vi "Build DAQmx Settings.vi"(7 "Host Resources":T10, 11 "Hardware Configuration in":T1) -> (0 "DAQ Task Kinds":string[](array[string]), 1 "Physical Channels":string[](array[string]), 3 "Hardware Configuration in out":T1, 4 "DAQ Device Names":string[](array[string]))   [LabVIEW 2021, in "Load Frame.lvlib"]
doc: "Match the channel settings in 'Hardware Configuration in' with IO devices available in 'Host Resources' and return the selected devices, their physical channels, and corresponding DAQmx Task kind (like AI or AO or Counter)."
uses:
  Load Frame.lvlib
  Acquisition/Hardware Configuration.ctl
  Acquisition/Channel Settings.ctl
  Acquisition/IO Device.ctl
  Acquisition/Sensor Type.ctl
  Interval Timer/Repeat Interval.ctl
  Interval Timer/Interval Length.ctl
  Interval Timer/Interval Token.ctl
  Acquisition/IO Context.ctl
  Acquisition/IO API.ctl
  Acquisition/Host Resources.ctl
  Acquisition/Host Software Package.ctl
  Acquisition/Host IO Resource.ctl
  Acquisition/Acquisition.lvlib
  Interval Timer/Interval Timer.lvlib
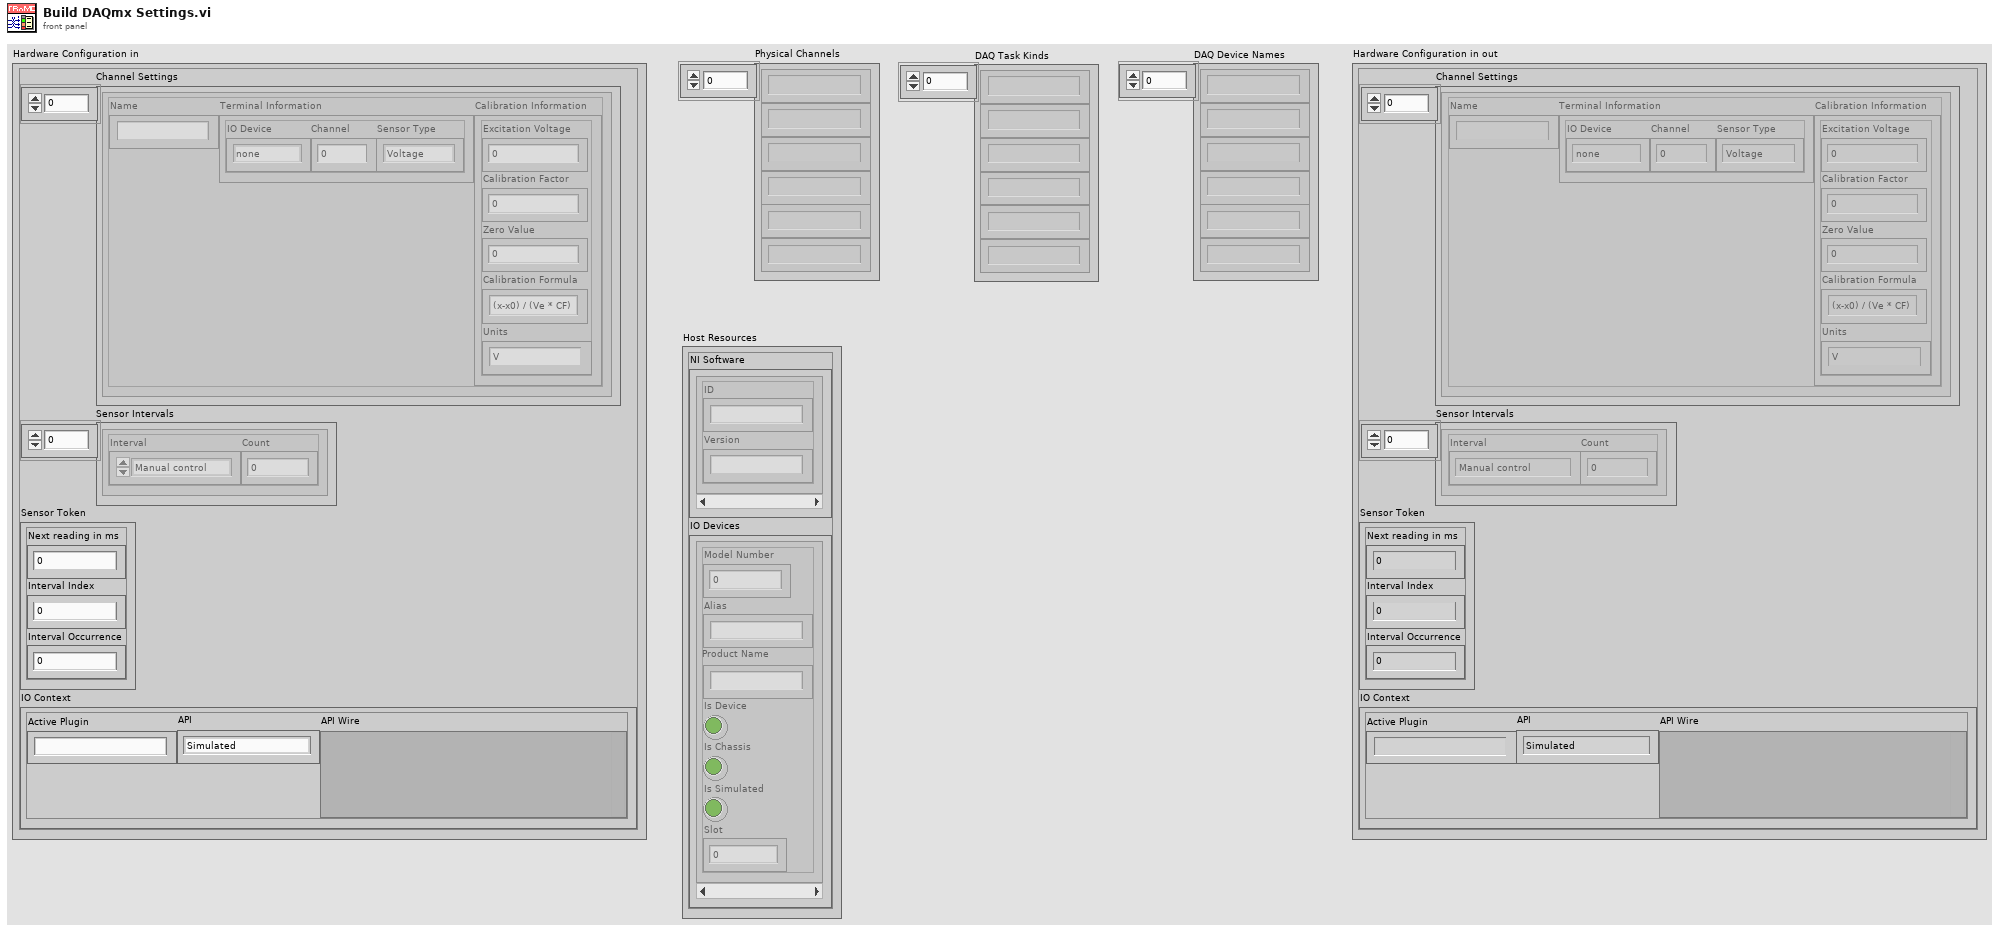
[diagram p1: front panel]
types:
  T1 = typedef "Acquisition.lvlib/Hardware Configuration.ctl" = cluster{"Channel Settings":T2[], "Sensor Intervals":T5[], "Sensor Token":T7, "IO Context":T8}
  T2 = typedef "Acquisition.lvlib/Channel Settings.ctl" = cluster{"Name":string, "Terminal Information":cluster{"IO Device":T3, "Channel":i32, "Sensor Type":T4}, "Calibration Information":cluster{"Excitation Voltage":dbl, "Calibration Factor":dbl, "Zero Value":dbl, "Calibration Formula":string, "Units":string}}
  T3 = typedef "Acquisition.lvlib/IO Device.ctl" = enum16{"none", "9219", "9401"}
  T4 = typedef "Acquisition.lvlib/Sensor Type.ctl" = enum16{"Voltage", "Load", "Pressure", "Encoder"}
  T5 = typedef "Interval Timer.lvlib/Repeat Interval.ctl" = cluster{"Interval":T6, "Count":i32}
  T6 = typedef "Interval Timer.lvlib/Interval Length.ctl" = enum16{"Manual control", "1 second", "10 seconds", "30 seconds", "60 seconds", "600 seconds", "1200 seconds", "3600 seconds"}
  T7 = typedef "Interval Timer.lvlib/Interval Token.ctl" = cluster{"Next reading in ms":u32, "Interval Index":i32, "Interval Occurrence":i32}
  T8 = typedef "Acquisition.lvlib/IO Context.ctl" = cluster{"Active Plugin":string, "API":T9, "API Wire":variant}
  T9 = typedef "Acquisition.lvlib/IO API.ctl" = enum16{"Simulated", "DAQmx"}
  T10 = typedef "Acquisition.lvlib/Host Resources.ctl" = cluster{"NI Software":T11[], "IO Devices":T12[]}
  T11 = typedef "Acquisition.lvlib/Host Software Package.ctl" = cluster{"ID":string, "Version":string}
  T12 = typedef "Acquisition.lvlib/Host IO Resource.ctl" = cluster{"Model Number":u32, "Alias":string, "Product Name":string, "Is Device":bool, "Is Chassis":bool, "Is Simulated":bool, "Slot":i32}
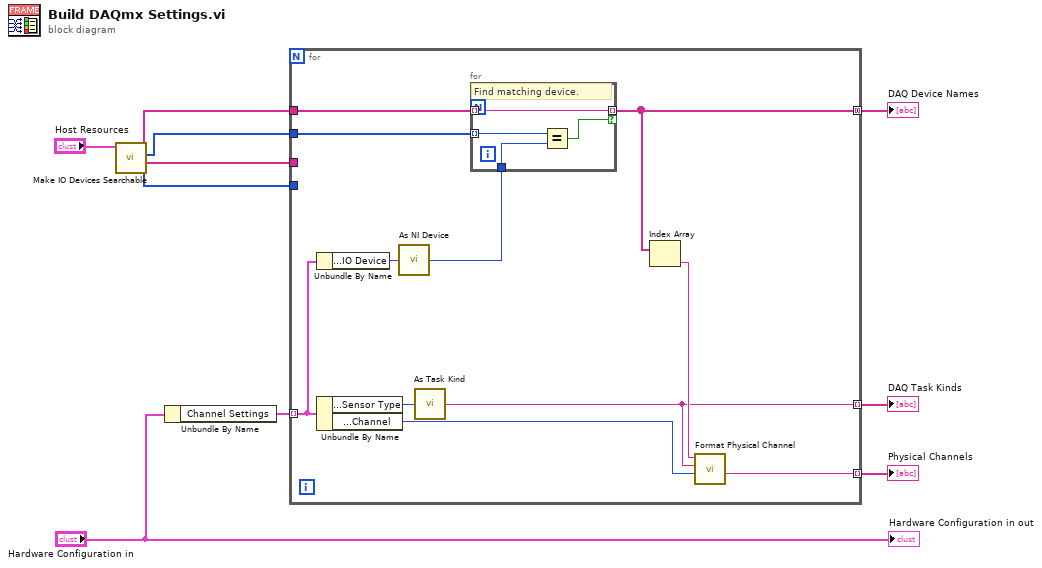
[diagram p0: block diagram]
diagram:
  n1 = call "Make IO Devices Searchable.vi"("Host Resources"="Host Resources") -> ("By Slot"=w4:i32[], "By Product Name"=w5:string[], "By Model Number"=w6:u32[], "By Alias"=w7:string[])  [unwired: 7 in]
  n2 = Unbundle By Name("Hardware Configuration in") -> ("Channel Settings"=w9:T2[])
  n3 = for {
    tunnel: w9 -> [w17] mode=indexing
    tunnel: w7 -> [w21]
    tunnel: w6 -> [w18]
    tunnel: w5 -> [_]
    tunnel: w4 -> [_]
    tunnel: [w15] -> w3 mode=concatenating
    tunnel: [w12] -> w2 mode=indexing
    tunnel: [w14] -> w1 mode=indexing
    n4 = Unbundle By Name(w17) -> ("Terminal Information.IO Device"=w20:T3)
    n5 = Unbundle By Name(w17) -> ("Terminal Information.Sensor Type"=w16:T4, "Terminal Information.Channel"=w11:i32)
    n6 = call "As NI Device.vi"("IO Device"=w20) -> ("As NI Device"=w19:i32)
    n7 = call "As Task Kind.vi"("Sensor Type"=w16) -> ("DAQmx Task prefix"=w12:string)
    n8 = for {
      tunnel: w21 -> [w22] mode=indexing
      tunnel: w19 -> [w24]
      tunnel: w18 -> [w23] mode=indexing
      tunnel: [w22] -> w15 mode=indexing if=w25
      # "Find matching device."
      n9 = Equal?(x=w23, y=w24) -> (x = y?=w25:bool)
    }
    n10 = Index Array(array=w15) -> (element=w13:string)  [unwired: 1 in]
    n11 = call "Format Physical Channel.vi"("Channel"=w11, "DAQmx Task prefix"=w12, "Alias"=w13) -> ("Physical Channel"=w14:string)  [unwired: 8 in]
  }
  "DAQ Device Names" <- w3
  "DAQ Task Kinds" <- w2
  "Physical Channels" <- w1
  "Hardware Configuration in out" <- "Hardware Configuration in"
